vi "ATF-Pump-Sequence AI Collector FGV.vi"(0 "Value":dbl, 1 "Option":T2(ring), 5 "Values":dbl[](array[numeric])=[0.0, 0.0, 0.0, 0.0, 0.0, 0.0, 0.0, 0.0], 7 "Loop":T1 items=["PT 1", "PT 2", "PT 3", "PT 4", "PT 5", "PT 6"], 9 "Loops":T1[](array[typedef]) items=["PT 1", "PT 2", "PT 3", "PT 4", "PT 5", "PT 6"], 11 "error in (no error)":errorcluster) -> (4 "Value Out":dbl, 10 "Values List Out":dbl[](array[numeric]), 15 "error out":errorcluster)   [LabVIEW 2022 SP3]
uses:
  RT Controls/AI Names.ctl
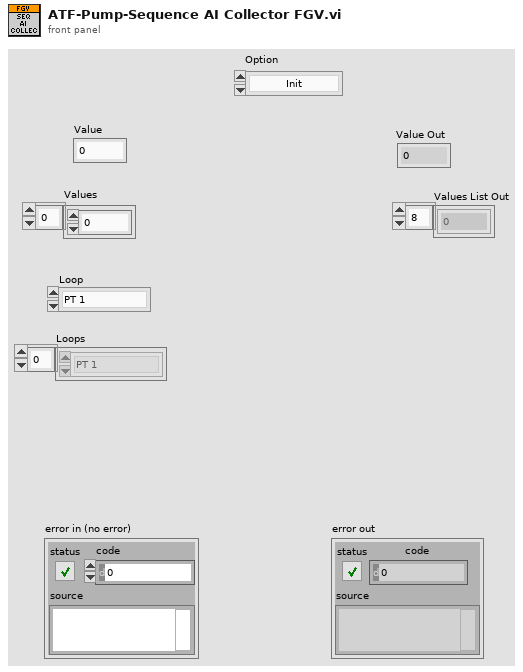
[diagram p1: front panel]
types:
  T1 = typedef "AI Names.ctl" = u16
  T2 = enum16{"Init", "Read 'All'", "Read 'n'", "Read '1'", "Write '1'", "Write 'n'", "Write 'All'"}
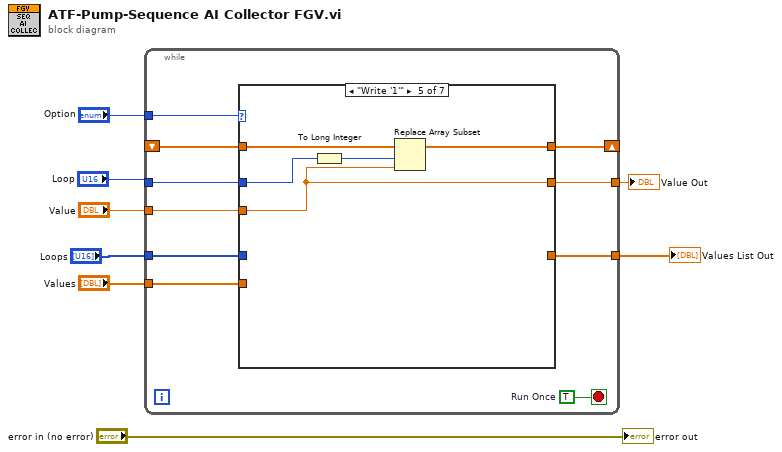
[diagram p0: block diagram]
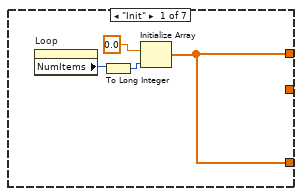
[diagram p2: hidden frame]
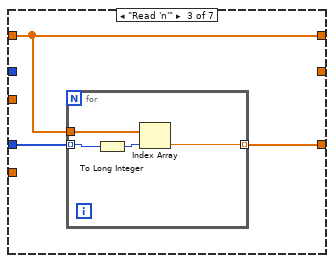
[diagram p4: hidden frame]
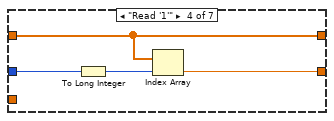
[diagram p5: hidden frame]
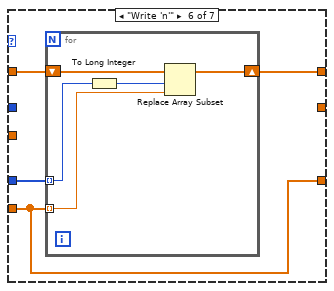
[diagram p6: hidden frame]
diagram:
  n1 = while {
    tunnel: "Option" -> [w17]
    shift-right: [w16] -> _
    shift-left: _ -> [w15]
    tunnel: "Loops" -> [w14]
    tunnel: [w13] -> w7
    tunnel: "Loop" -> [w12]
    tunnel: [w11] -> w6
    tunnel: "Value" -> [w10]
    tunnel: "Values" -> [w9]
    stop <- w18 stop-if-true
    w18 = TRUE  # Run Once
    n2 = case shown="\"Write '1'\"" w17 {
      tunnel: [w22 w23 w25 w34 w38 w42 w49] -> w16
      tunnel: w15 -> [_ w23 w25 w34 w39 w43 _]
      tunnel: w14 -> [_ _ w26 _ _ w41 _]
      tunnel: [w22 w23 w24 _ _ w40 w49] -> w13
      tunnel: w12 -> [_ _ _ w33 w37 _ _]
      tunnel: [_ _ _ w32 w36 _ _] -> w11
      tunnel: w10 -> [_ _ _ _ w36 _ _]
      tunnel: w9 -> [_ _ _ _ _ w40 w49]
      frame "Init" {
        n3 = property on="Loop" class="Ring (strict)"() -> ("NumItems"=w20:u32)  [unwired: 2 in, 2 out]
        n4 = To Long Integer(number=w20) -> (32bit integer=w21:i32)
        n5 = Initialize Array(0.0 ("Value"), w21) -> (w22:dbl[])
      }
      frame "Read 'All'", Default {
      }
      frame "Read 'n'" {
        n6 = for {
          tunnel: w26 -> [w28] mode=indexing
          tunnel: w25 -> [w30]
          tunnel: [w29] -> w24 mode=indexing
          n7 = To Long Integer(number=w28) -> (32bit integer=w27:i32)
          n8 = Index Array(array=w30, index=w27) -> (element=w29:dbl)
        }
      }
      frame "Read '1'" {
        n9 = To Long Integer(number=w33) -> (32bit integer=w31:i32)
        n10 = Index Array(array=w34, index=w31) -> (element=w32:dbl)
      }
      frame "Write '1'" {
        n11 = To Long Integer(number=w37) -> (32bit integer=w35:i32)
        n12 = Replace Array Subset(array=w39, new element=w36, index=w35) -> (w38:dbl[])
      }
      frame "Write 'n'" {
        n13 = for {
          tunnel: w41 -> [w46] mode=indexing
          tunnel: w40 -> [w45] mode=indexing
          shift-right: [w47] -> w42
          shift-left: w43 -> [w48]
          n14 = To Long Integer(number=w46) -> (32bit integer=w44:i32)
          n15 = Replace Array Subset(array=w48, new element=w45, index=w44) -> (w47:dbl[])
        }
      }
      frame "Write 'All'" {
      }
    }
  }
  "Values List Out" <- w7
  "Value Out" <- w6
  "error out" <- "error in (no error)"
